vi "DSF.Shared.Configuration.Transfer.Initialize.vi"(7 "direction":T1, 8 "error in (no error)":errorcluster, 10 "Transfer Configuration cluster":T2, 11 "Transfer Configuration in":refnum<class "VeriStand DSF.Transfer.Configuration.lvclass">) -> (0 "error out":errorcluster, 3 "Transfer Configuration out":refnum<class "VeriStand DSF.Transfer.Configuration.lvclass">)   [LabVIEW 2017, in "Data Sharing Framework Engine.lvlib" / "VeriStand DSF.Transfer.Configuration.lvclass"]
uses:
  VeriStand DSF.Transfer.Configuration.lvclass
  DSF Core/Built/Windows/Engine/DSF.Engine.lvlibp/DSF Configuration API/1.0.0/Public/Controls/DSF Engine Transfer Configuration.ctl
  DSF Core/Built/Windows/Engine/DSF.Engine.lvlibp/DSF Configuration API/1.0.0/Public/Controls/DSF Byte Order.ctl
  DSF Core/Built/Windows/Engine/DSF.Engine.lvlibp/DSF Configuration API/1.0.0/Public/Controls/DSF Engine Channel Configuration.ctl
  DSF Core/Built/Windows/Engine/DSF.Engine.lvlibp/DSF Configuration API/1.0.0/Public/Controls/DSF Data Type.ctl
  DSF Core/Built/Windows/Engine/DSF.Engine.lvlibp/DSF Configuration API/1.0.0/Public/Controls/DSF Settings Info.ctl
  DSF Core/Built/Windows/Engine/DSF.Engine.lvlibp/DSF Configuration API/1.0.0/Public/Controls/DSF Direction.ctl
  <vilib>/NI Veristand/Custom Device API/Custom Device Channel Type.ctl
  <vilib>/NI Veristand/Custom Device API/Data Access Type.ctl
  VeriStand DSF.Transfer.Configuration.lvclass/VeriStand DSF.Transfer.Configuration.ctl
  DSF Core/Built/Windows/Engine/DSF.Engine.lvlibp/Shared/Classes/Transfer/DSF.Shared.Configuration.Transfer.lvclass
  <vilib>/NI Veristand/Custom Device API/Custom Device API.lvlib
  DSF Core/Built/Windows/Engine/DSF.Engine.lvlibp/DSF Configuration API/1.0.0/DSF Configuration API.lvlib
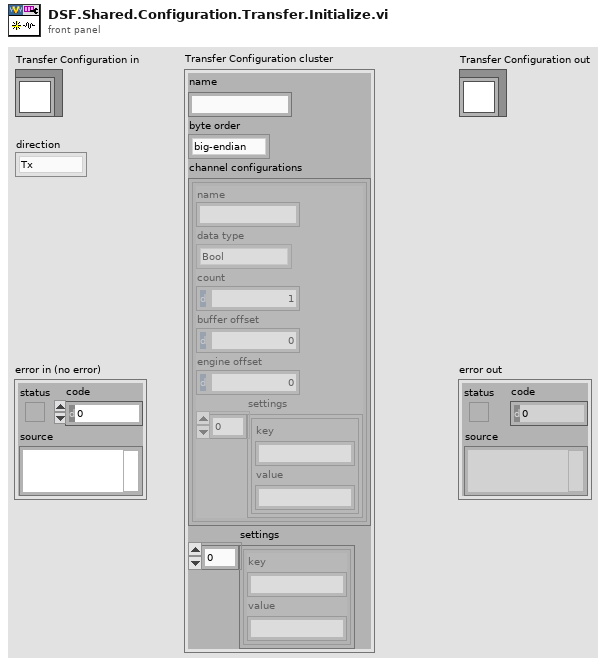
[diagram p1: front panel]
types:
  T1 = typedef "DSF.Engine.lvlibp/DSF Configuration API.lvlib/DSF Direction.ctl" = enum8{"Tx", "Rx"}
  T2 = typedef "DSF.Engine.lvlibp/DSF Configuration API.lvlib/DSF Engine Transfer Configuration.ctl" = cluster{"name":string, "byte order":T3, "channel configurations":T4[], "settings":T6}
  T3 = typedef "DSF.Engine.lvlibp/DSF Configuration API.lvlib/DSF Byte Order.ctl" = enum8{"big-endian", "little-endian"}
  T4 = typedef "DSF.Engine.lvlibp/DSF Configuration API.lvlib/DSF Engine Channel Configuration.ctl" = cluster{"name":string, "data type":T5, "count":u64, "buffer offset":u64, "engine offset":u64, "settings":T6}
  T5 = typedef "DSF.Engine.lvlibp/DSF Configuration API.lvlib/DSF Data Type.ctl" = enum8{"Bool", "SGL", "DBL", "I8", "I16", "I32", "I64", "U8", "U16", "U32", "U64"}
  T6 = typedef "DSF.Engine.lvlibp/DSF Configuration API.lvlib/DSF Settings Info.ctl" = cluster{"key":string, "value":string}[]
  T7 = typedef "Custom Device API.lvlib/Data Access Type.ctl" = enum16{"Read", "Write"}
  T8 = typedef "Custom Device API.lvlib/Custom Device Channel Type.ctl" = enum16{"Input", "Output"}
  T9 = typedef "Custom Device API.lvlib/Custom Device Item Ref.ctl" = u64
  T10 = typedef "Custom Device API.lvlib/Data Reference.ctl" = i32
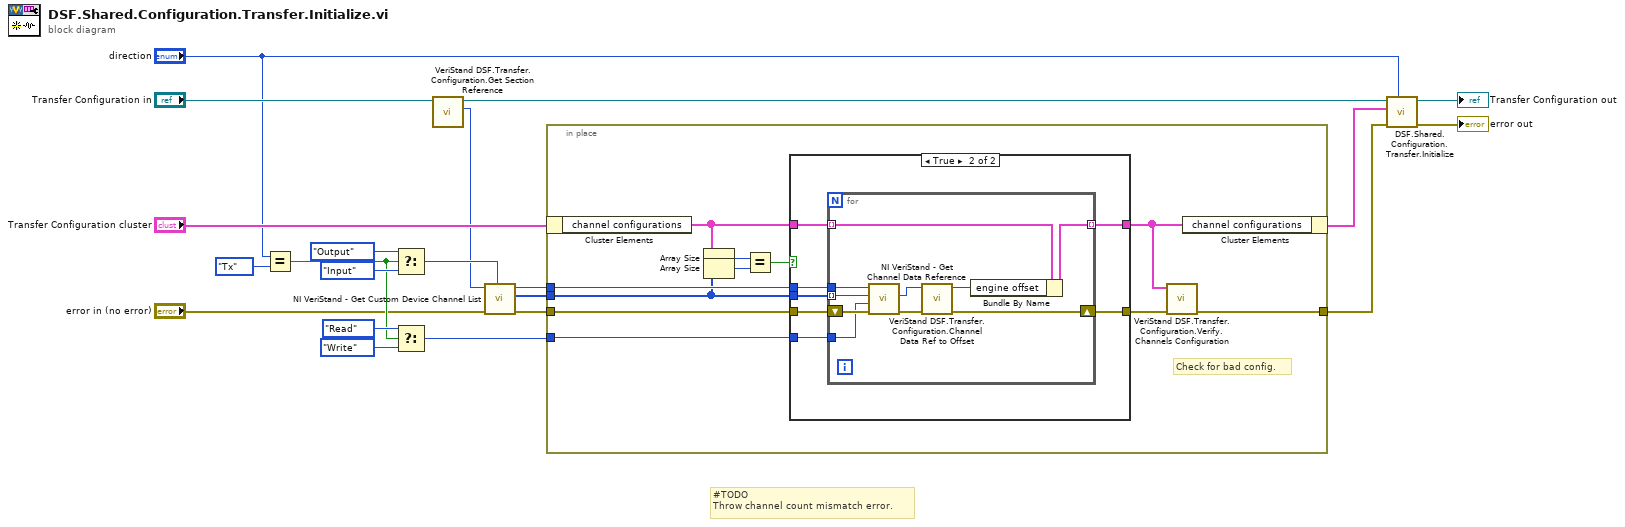
[diagram p0: block diagram]
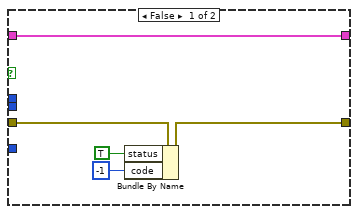
[diagram p2: hidden frame]
diagram:
  # "#TODO\nThrow channel count mismatch error."
  n1 = Equal?(x="direction", y=DSF_Direction."Tx") -> (x = y?=w10:bool)
  n2 = Select(t=Custom_Device_Channel_Type."Output" ("Channel Type"), s=w10, f=Custom_Device_Channel_Type."Input" ("Channel Type")) -> (s? t:f=w17:T8)
  n3 = Select(t=Data_Access_Type."Read" ("Access"), s=w10, f=Data_Access_Type."Write" ("Access")) -> (s? t:f=w11:T7)
  n4 = call "VeriStand DSF.Transfer.Configuration.Get Section Reference.vi"("VeriStand DSF.Transfer.Configuration in"="Transfer Configuration in") -> ("Section Ref"=w6:T9, "VeriStand DSF.Transfer.Configuration out"=w3:refnum<class "VeriStand DSF.Transfer.Configuration.lvclass">)  [unwired: 9 in]
  n5 = call <vilib>:"NI VeriStand - Get Custom Device Channel List.vi"("Channel Type"=w17, "error in (no error)"="error in (no error)", "Device Ref in"=w6) -> ("error out"=w16:errorcluster, "Specified Channel Ref List"=w15:T9[], "Device Ref out"=w14:T9)  [unwired: 6 in]
  n6 = in-place {
    in-place-border: w16 -> [w30]
    in-place-border: w15 -> [w25]
    in-place-border: w14 -> [w28]
    in-place-border: w11 -> [w27]
    in-place-border: [w22] -> w1
    # "Check for bad config."
    n7 = in-place-cluster #1("Transfer Configuration cluster") -> ("channel configurations"=w26:T4[])
    n8 = Array Size(array=w26) -> (size(s)=w31:i32)
    n9 = Array Size(array=w25) -> (size(s)=w32:i32)
    n10 = Equal?(x=w31, y=w32) -> (x = y?=w29:bool)
    n11 = case shown="True" w29 {
      tunnel: w30 -> [w37 w44]
      tunnel: [w36 w43] -> w24
      tunnel: w25 -> [_ w42]
      tunnel: w28 -> [_ w40]
      tunnel: w27 -> [_ w41]
      tunnel: w26 -> [w34 w39]
      tunnel: [w34 w38] -> w23
      frame False {
        n12 = Bundle By Name(cluster=w37, "status"=TRUE, "code"=-1) -> (w36:errorcluster)
      }
      frame True {
        n13 = for {
          tunnel: w42 -> [w53] mode=indexing
          shift-right: [w49] -> w43
          shift-left: w44 -> [w54]
          tunnel: w41 -> [w51]
          tunnel: w40 -> [w52]
          tunnel: w39 -> [w46] mode=indexing
          tunnel: [w45] -> w38 mode=indexing
          n14 = call <vilib>:"NI VeriStand - Get Channel Data Reference.vi"("error in (no error)"=w54, "Access"=w51, "Channel Ref in"=w53, "Device Ref in"=w52) -> ("error out"=w50:errorcluster, "Channel Data Reference"=w48:T10)  [unwired: 6 out]
          n15 = call "VeriStand DSF.Transfer.Configuration.Channel Data Ref to Offset.vi"("error in (no error)"=w50, "Channel Data Reference"=w48) -> ("error out"=w49:errorcluster, "channel offset"=w47:u64)  [unwired: 8 in]
          n16 = Bundle By Name(cluster=w46, "engine offset"=w47) -> (w45:T4)
        }
      }
    }
    n17 = call "VeriStand DSF.Transfer.Configuration.Verify.Channels Configuration.vi"("error in (no error)"=w24, "channel configurations"=w23) -> ("error out"=w22:errorcluster)  [unwired: 9 in]
    n18 = in-place-cluster #1("channel configurations"=w23) -> (w4:T2)
  }
  n19 = call-parent "DSF.Shared.Configuration.Transfer.Initialize.vi"("direction"="direction", "error in (no error)"=w1, "Transfer Configuration cluster"=w4, "Transfer Configuration in"=w3) -> ("error out"=→"error out":errorcluster, "Transfer Configuration out"=→"Transfer Configuration out":refnum<class "VeriStand DSF.Transfer.Configuration.lvclass">)  [unwired: 6 in]
